vi "Read and Parse Input File.vi"(0 "Input Parsed":T1, 5 "Directory Path":path=path "C:/Soliton Premier League 2015/Battle Field/Dragon Tamers", 7 "Play Number":i32, 11 "error in (no error)":errorcluster) -> (4 "Input Parsed":T1, 15 "error out":errorcluster)   [LabVIEW 2014, in "Dragon Tamers.lvlib"]
uses:
  Dragon Tamers.lvlib
  Typedefs/Input Parsed.ctl
  Typedefs/King.ctl
  Typedefs/Cell Pos.ctl
  Typedefs/Board.ctl
  Typedefs/Board Cell.ctl
  Typedefs/Cell Occupancy.ctl
panel:
  out "Array":string[](array[string])
  out "File Contents":string
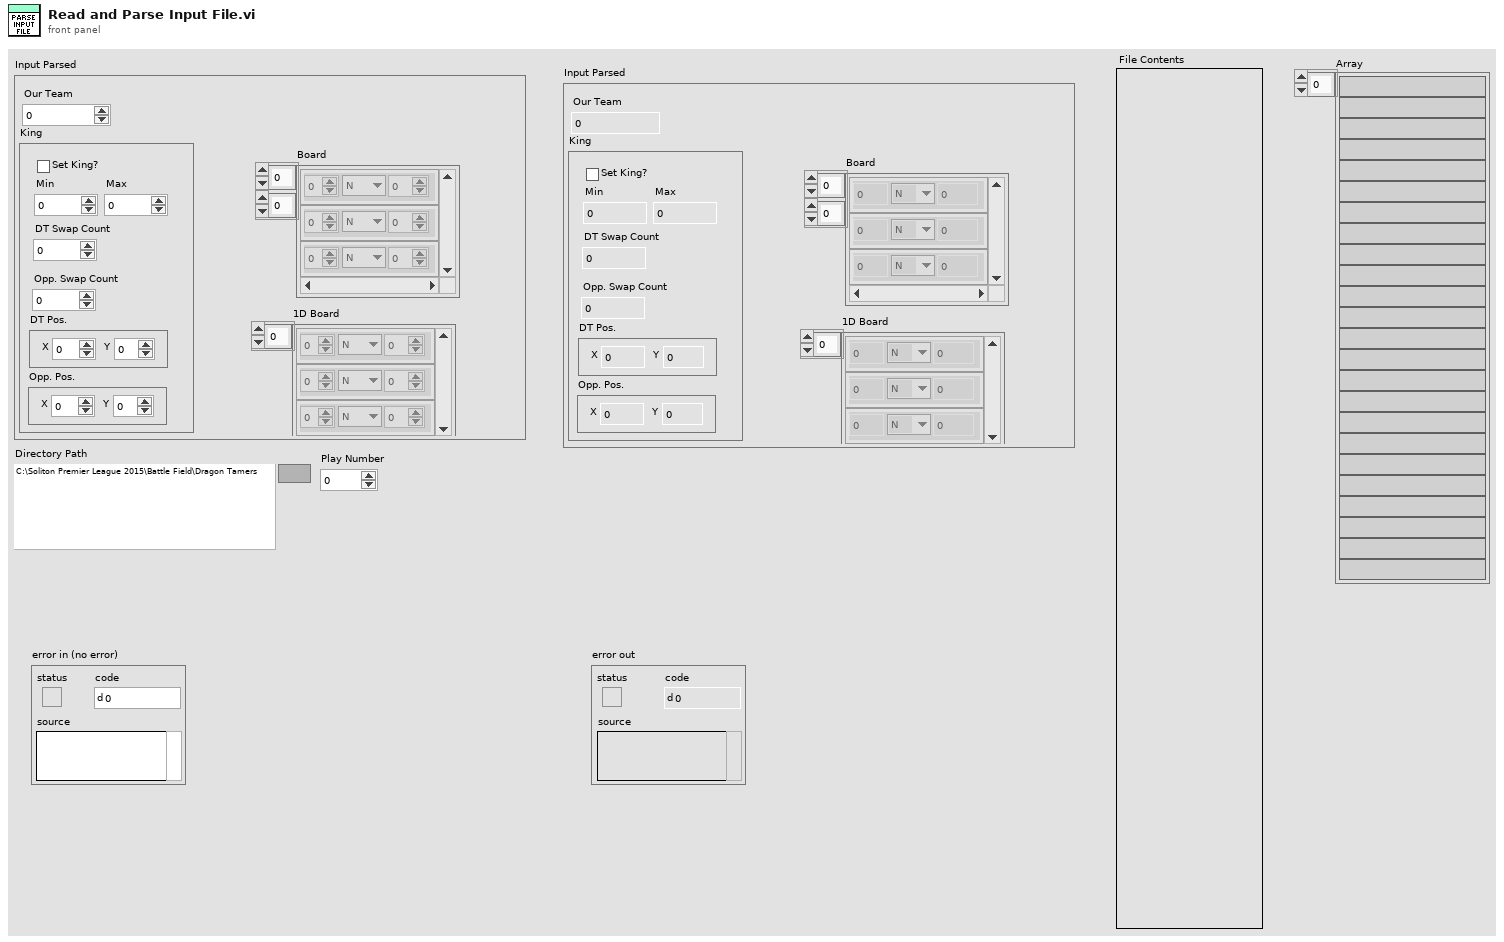
[diagram p1: front panel]
types:
  T1 = typedef "Dragon Tamers.lvlib/Input Parsed.ctl" = cluster{"Our Team":i32, "King":T2, "Board":T4, "1D Board":T5[]}
  T2 = typedef "Dragon Tamers.lvlib/King.ctl" = cluster{"Set King?":bool, "Min":i32, "Max":i32, "DT Swap Count":i32, "Opp. Swap Count":i32, "DT Pos.":T3, "Opp. Pos.":T3}
  T3 = typedef "Dragon Tamers.lvlib/Cell Pos.ctl" = cluster{"X":i32, "Y":i32}
  T4 = typedef "Dragon Tamers.lvlib/Board.ctl" = T5[][]
  T5 = typedef "Dragon Tamers.lvlib/Board Cell.ctl" = cluster{"Team":i32, "Occu.":T6, "Count":i32}
  T6 = typedef "Dragon Tamers.lvlib/Cell Occupancy.ctl" = enum16{"N", "C", "K"}
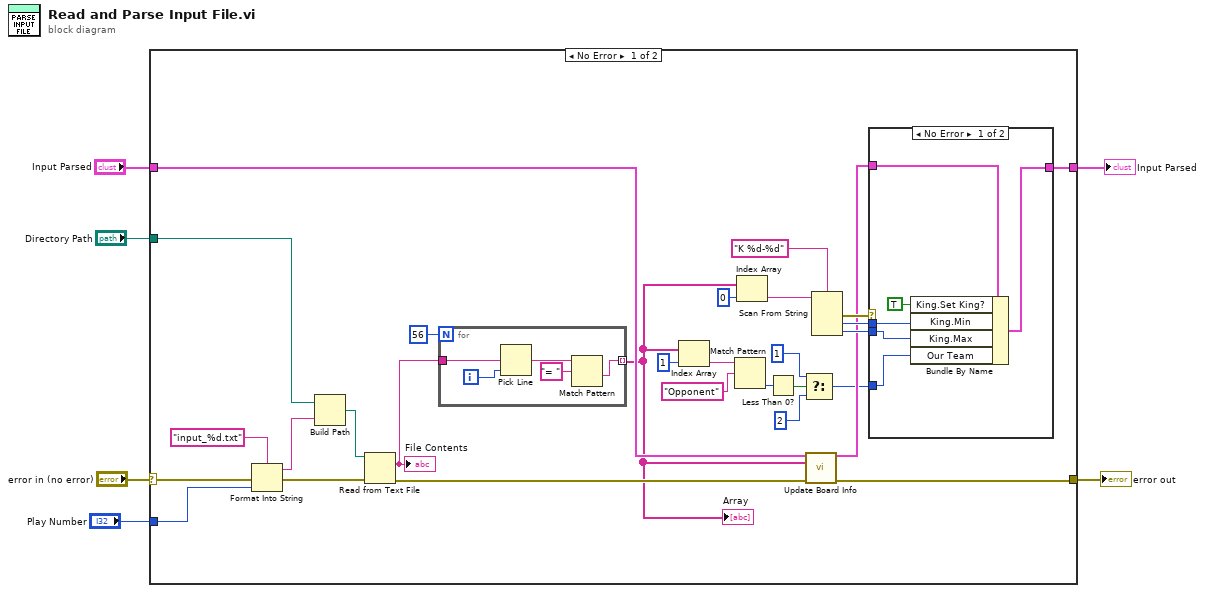
[diagram p0: block diagram]
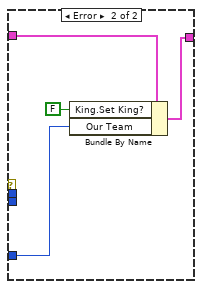
[diagram p2: hidden frame]
diagram:
  n1 = case shown="No Error" "error in (no error)" {
    selector: "error in (no error)" -> [w35 w52]
    tunnel: [w21 w52] -> w5
    tunnel: "Directory Path" -> [w32 _]
    tunnel: "Play Number" -> [w34 _]
    tunnel: "Input Parsed" -> [w20 w51]
    tunnel: [w16 w51] -> w1
    frame No Error {
      n2 = Format Into String(format string="input_%d.txt", error in=w35, w34) -> (resulting string=w31:string, error out=w30:errorcluster)  [unwired: 1 in]
      n3 = Build Path(base path=w32, name or relative path=w31) -> (appended path=w29:path)
      n4 = Read from Text File(file (use dialog)=w29, error in=w30) -> (text=w27:string, error out=w22:errorcluster)  [unwired: 2 in, 2 out]
      "File Contents" <- w27
      n5 = for {
        N: 56 -> [_]
        tunnel: w27 -> [w50]
        tunnel: [w46] -> w15 mode=indexing
        i -> [w49]
        n6 = Pick Line(multi-line string=w50, line index=w49) -> (output string=w47:string)  [unwired: 1 in]
        n7 = Match Pattern(string=w47, regular expression="= ") -> (after substring=w46:string)  [unwired: 1 in, 3 out]
      }
      "Array" <- w15
      n8 = Index Array(array=w15, index=1) -> (element=w13:string)
      n9 = Match Pattern(string=w13, regular expression="Opponent") -> (offset past match=w11:i32)  [unwired: 1 in, 3 out]
      n10 = Index Array(array=w15, index=0) -> (element=w25:string)
      n11 = Less Than 0?(x=w11) -> (x < 0?=w10:bool)
      n12 = Select(t=1, s=w10, f=2) -> (s? t:f=w7:i32)
      n13 = call "Update Board Info.vi"("Input Parsed"=w20, "Array"=w15, "error in (no error)"=w22) -> ("Input Parsed"=w17:T1, "error out"=w21:errorcluster)  [unwired: 11 in]
      n14 = Scan From String(format string="K %d-%d", input string=w25) -> (error out=w23:errorcluster, output 1=w19:i32, output 2=w18:i32)  [unwired: 4 in, 2 out]
      n15 = case shown="No Error" w23 {
        tunnel: w19 -> [w39 _]
        tunnel: w18 -> [w38 _]
        tunnel: w17 -> [w41 w45]
        tunnel: [w37 w44] -> w16
        tunnel: w7 -> [w36 w42]
        frame No Error {
          n16 = Bundle By Name(cluster=w41, "King.Set King?"=TRUE, "King.Min"=w39, "King.Max"=w38, "Our Team"=w36) -> (w37:T1)
        }
        frame Error {
          n17 = Bundle By Name(cluster=w45, "King.Set King?"=FALSE, "Our Team"=w42) -> (w44:T1)
        }
      }
    }
    frame Error {
    }
  }
  "error out" <- w5
  "Input Parsed" <- w1
